vi "Initialize Owner Attribute.vi"(9 "Shared Key":string, 10 "Owner GUID":string, 11 "Owner Name":string) -> (3 "Attribute.Owner":refnum<class "Attribute.Owner.lvclass">)   [LabVIEW 2019, in "Attribute.Owner.lvclass"]
doc: "JKI State Machine Objects (SMO) 1.3.0.56\nJKI - JKI\nCopyright (c) 2017, JKI"
uses:
  Attribute.Owner.lvclass
  Packet -- Cluster.ctl
  Attribute.Owner.lvclass/Attribute.Owner.ctl
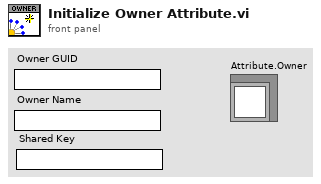
[diagram p1: front panel]
types:
  T1 = typedef "Attribute.Owner.lvclass/Packet -- Cluster.ctl" = cluster{"Message":string, "Payload":variant, "Source GUID":string}
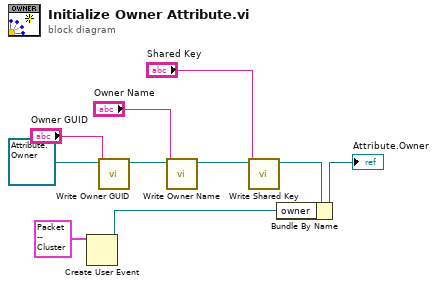
[diagram p0: block diagram]
diagram:
  n1 = Create User Event(user event datatype=T1 {"Message"="", "Payload"=variant, "Source GUID"=""} ("Packet")) -> (user event=w3:refnum<user-event>)  [unwired: 1 in, 1 out]
  n2 = call "Write Owner GUID.vi"("Owner GUID"="Owner GUID", "Attribute.Owner in"=refnum<class "Attribute.Owner.lvclass"> refnum) -> ("Attribute.Owner out"=w9:refnum<class "Attribute.Owner.lvclass">)  [unwired: 8 in, 1 out]
  n3 = call "Write Owner Name.vi"("Owner Name"="Owner Name", "Attribute.Owner in"=w9) -> ("Attribute.Owner out"=w8:refnum<class "Attribute.Owner.lvclass">)  [unwired: 8 in, 1 out]
  n4 = call "Write Shared Key.vi"("Shared Key"="Shared Key", "Attribute.Owner in"=w8) -> ("Attribute.Owner out"=w2:refnum<class "Attribute.Owner.lvclass">)  [unwired: 8 in, 1 out]
  n5 = Bundle By Name(cluster=w2, "owner"=w3) -> (→"Attribute.Owner":refnum<class "Attribute.Owner.lvclass">)
